vi "Append to Change Log.vi"(8 "error in (no error)":errorcluster, 9 "Release Notes":string, 10 "selected path":path) -> (0 "error out":errorcluster, 2 "VI Package Build Spec Data":T1)   [LabVIEW 2019, in "VIPM.lvlib"]
uses:
  <vilib>/JKI/VIPM API/command-line/support/VI Package Build Spec Data Cluster_vipm_api.ctl
  <vilib>/JKI/VIPM API/command-line/support/Version Info Cluster_vipm_api.ctl
  VIPM.lvlib
  <vilib>/JKI/VIPM API/VIPM API_vipm_api.lvlib
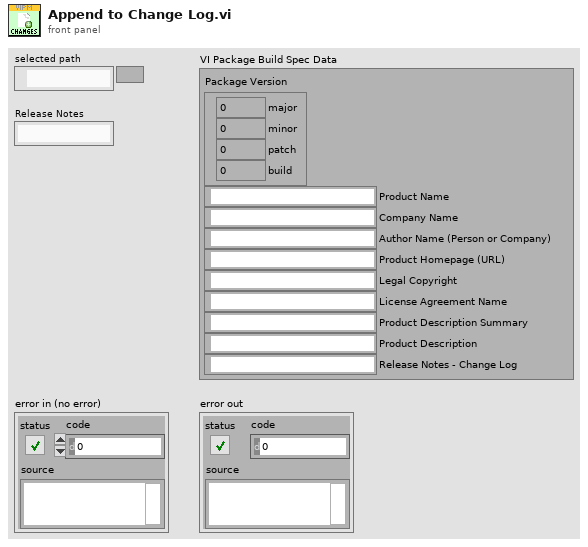
[diagram p1: front panel]
types:
  T1 = typedef "VIPM API_vipm_api.lvlib/VI Package Build Spec Data Cluster_vipm_api.ctl" = cluster{"Package Version":T2, "Product Name":string, "Company Name":string, "Author Name (Person or Company)":string, "Product Homepage (URL)":string, "Legal Copyright":string, "License Agreement Name":string, "Product Description Summary":string, "Product Description":string, "Release Notes - Change Log":string}
  T2 = typedef "VIPM API_vipm_api.lvlib/Version Info Cluster_vipm_api.ctl" = cluster{"major":u32, "minor":u32, "patch":u32, "build":u32}
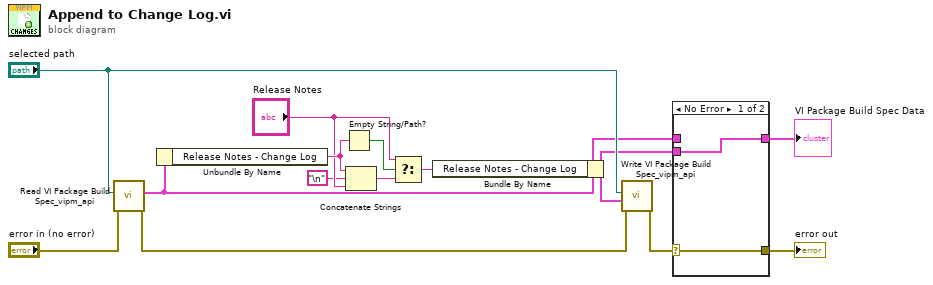
[diagram p0: block diagram]
diagram:
  n1 = call <vilib>:"Read VI Package Build Spec_vipm_api.vi"("error in (no error)"="error in (no error)", "Path to VIPB File"="selected path") -> ("error out"=w7:errorcluster, "VI Package Build Spec Data"=w2:T1)  [unwired: 8 in]
  n2 = Unbundle By Name(w2) -> ("Release Notes - Change Log"=w13:string)
  n3 = Empty String/Path?(string/path=w13) -> (empty?=w9:bool)
  n4 = Concatenate Strings(w13, "\n", "Release Notes") -> (w14:string)
  n5 = Select(t="Release Notes", s=w9, f=w14) -> (s? t:f=w10:string)
  n6 = Bundle By Name(cluster=w2, "Release Notes - Change Log"=w10) -> (w1:T1)
  n7 = call <vilib>:"Write VI Package Build Spec_vipm_api.vi"("error in (no error)"=w7, "VI Package Build Spec Data"=w1, "Path to VIPB File"="selected path") -> ("error out"=w5:errorcluster)  [unwired: 8 in]
  n8 = case shown="No Error" w5 {
    selector: w5 -> [w16 w18]
    tunnel: [w16 w18] -> w4
    tunnel: [w15 w17] -> w3
    tunnel: w2 -> [_ w17]
    tunnel: w1 -> [w15 _]
    frame No Error {
    }
    frame Error {
    }
  }
  "error out" <- w4
  "VI Package Build Spec Data" <- w3
